vi "Voltage Interrupt.vi"(9 "AnalogTriggerSource":T1={"DevStatus"={"status"=FALSE, "code"=0, "source"=""}, "Controller"=enum."Controller 1", "Analog Channel"=enum."Invalid"}, 11 "Enum":T4) -> ()   [LabVIEW 2014]
uses:
  TypeDefs/SRE Enum.ctl
  <vilib>/Rock Robotics/WPI/AnalogChannel/WPI_AnalogChannelDevRef.ctl
  <vilib>/Rock Robotics/SystemInterfaces/Typedef/FPGA_TypedefAnalogModule.ctl
  <vilib>/Rock Robotics/SystemInterfaces/AI/FPGA_AIChannel.ctl
  <vilib>/Rock Robotics/WPI/Counter/WPI_CounterAnalogTriggerToDigitalSource.vi
  <vilib>/Rock Robotics/SystemInterfaces/CounterEncoderSourceConvertion/FPGA_CounterEncoderSourceConvertionLVSourceTypeToFPGAType.vi
  <vilib>/Rock Robotics/WPI/Interrupt/WPI_InterruptCache.vi
  <vilib>/Rock Robotics/SystemInterfaces/Interrupt/FPGA_InterruptWriteConfiguration.vi
  <vilib>/Rock Robotics/SystemInterfaces/Interrupt/FPGA_WaitOnInterrupt.vi
  <vilib>/Rock Robotics/WPI/Utilities/WPI_UtilitiesTimebaseConstants.vi
  <vilib>/Rock Robotics/SystemInterfaces/Interrupt/FPGA_InterruptReadTimestamp.vi
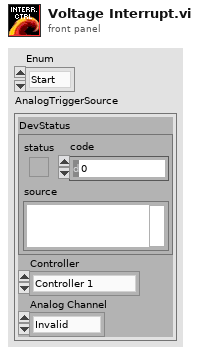
[diagram p1: front panel]
types:
  T1 = typedef "WPI_AnalogChannelDevRef.ctl" = cluster{"DevStatus":errorcluster, "Controller":T2, "Analog Channel":T3}
  T2 = typedef "FPGA_TypedefAnalogModule.ctl" = enum16{"Controller 1"}
  T3 = typedef "FPGA_AIChannel.ctl" = enum8{"AI 0", "AI 1", "AI 2", "AI 3", "AI MXP 0", "AI MXP 1", "AI MXP 2", "AI MXP 3", "Invalid"}
  T4 = typedef "SRE Enum.ctl" = enum16{"Start", "Run", "End"}
  T5 = typedef "FPGA_AnalogTriggerDevRef.ctl" = cluster{"DevStatus":errorcluster, "AnalogTriggerIndex":T6}
  T6 = typedef "FPGA_AnalogTriggerIndex.ctl" = enum8{"Trig 0", "Trig 1", "Trig 2", "Trig 3", "Trig 4", "Trig 5", "Trig 6", "Trig 7", "Invalid"}
  T7 = typedef "FPGA_CounterEncoderSourceConvertionLVSourceType.ctl" = cluster{"DevStatus":errorcluster, "AnalogTriggerMode?":bool, "DigitalMode":cluster{"Controller":T8, "DIO Channel":T9}, "AnalogTriggerMode":cluster{"AnalogTriggerIndex":T6, "OutputType":T10}}
  T8 = typedef "FPGA_TypedefDigitalModule.ctl" = enum16{"Controller 1"}
  T9 = typedef "FPGA_DIODigitalSourceChannel.ctl" = enum8{"DIO 0", "DIO 1", "DIO 2", "DIO 3", "DIO 4", "DIO 5", "DIO 6", "DIO 7", "DIO 8", "DIO 9", "DIO MXP 0", "DIO MXP 1", "DIO MXP 2", "DIO MXP 3", "DIO MXP 4", "DIO MXP 5", "DIO MXP 6", "DIO MXP 7", "DIO MXP 8", "DIO MXP 9", "DIO MXP 10", "DIO MXP 11", "DIO MXP 12", "DIO MXP 13", "DIO MXP 14", "DIO MXP 15", "Disabled"}
  T10 = typedef "FPGA_AnalogTriggerOutType.ctl" = enum16{"InWindow", "TriggerState", "Rising", "Falling"}
  T11 = typedef "WPI_InterruptRef.ctl" = cluster{"DevStatus":errorcluster, "InterruptIndex":T12}
  T12 = typedef "FPGA_InterruptIndex.ctl" = enum8{"0", "1", "2", "3", "4", "5", "6", "7", "Invalid"}
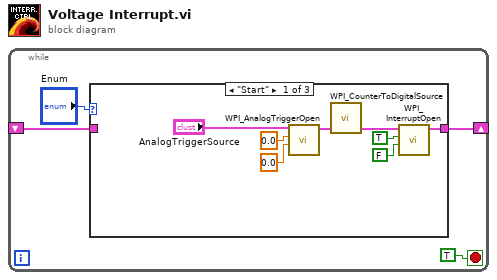
[diagram p0: block diagram]
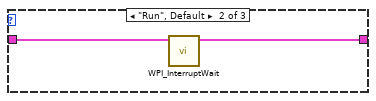
[diagram p2: hidden frame]
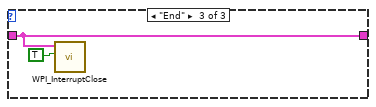
[diagram p3: hidden frame]
diagram:
  n1 = while {
    shift-right: [w2] -> _
    shift-left: _ -> [w3]
    stop <- TRUE stop-if-true
    n2 = case shown="\"Start\"" "Enum" {
      tunnel: w3 -> [_ w14 w16]
      tunnel: [w12 w13 w16] -> w2
      frame "Start" {
        n3 = call <vilib>:"WPI_AnalogTriggerOpen.vi"("LowerLimit (v)"=0.0, "UpperLimit (v)"=0.0, "AnalogTriggerSource"="AnalogTriggerSource") -> ("AnalogTriggerDevRef"=w10:T5)  [unwired: 7 in, 1 out]
        n4 = call-poly <vilib>:"WPI_CounterToDigitalSource.vi"("AnalogTriggerDevRef"=w10) -> ("Digital Source"=w11:T7)  [unwired: 6 in]
        n5 = call <vilib>:"WPI_InterruptOpen.vi"("Falling Edge"=FALSE, "Rising Edge"=TRUE, "Source"=w11) -> ("InterruptRef"=w12:T11)  [unwired: 7 in, 1 out]
      }
      frame "Run", Default {
        n6 = call <vilib>:"WPI_InterruptWait.vi"("InterruptRef"=w14) -> ("InterruptRef"=w13:T11)  [unwired: 6 in, 4 out]
      }
      frame "End" {
        n7 = call <vilib>:"WPI_InterruptClose.vi"("Close Dependencies"=TRUE, "InterruptRef"=w16) -> ()  [unwired: 9 in, 1 out]
      }
    }
  }
